vi "Enqueue - ClusterCommand.vi"(5 "Insert? (T)":bool=TRUE, 7 "At Front?":bool, 8 "error in (no error)":errorcluster, 10 "Command":string, 11 "Queue with Cluster Reference":T1) -> (0 "error out":errorcluster, 3 "Queue Out (dup)":T1)   [LabVIEW 2010]
doc: "This VI enqueues only the command portion of the cluster into the referenced queue.\n\nInputs:\nQueue with Cluster Reference - (queue) queue to insert cluster into\nCommand - (string) command part of the cluster to be inserted into the queue (may have arguments)\nAt Front? (F) - (bool) set TRUE to insert cluster at the beginning of the queue; FALSE (default) at the end\nInsert? (T) - (bool) TRUE = insert cluster into queue (default); FALSE = do not insert cluster (controlled via logic)\nerror in - error input cluster\n\nOutputs:\nQueue Out (dup) - (queue) duplicate reference to input queue\nerror out - error output cluster"
uses:
  <userlib>/Common/Queue with Cluster/TYP_Queue with Cluster Reference.ctl
panel:
  # "Inputs"
  # "Outputs"
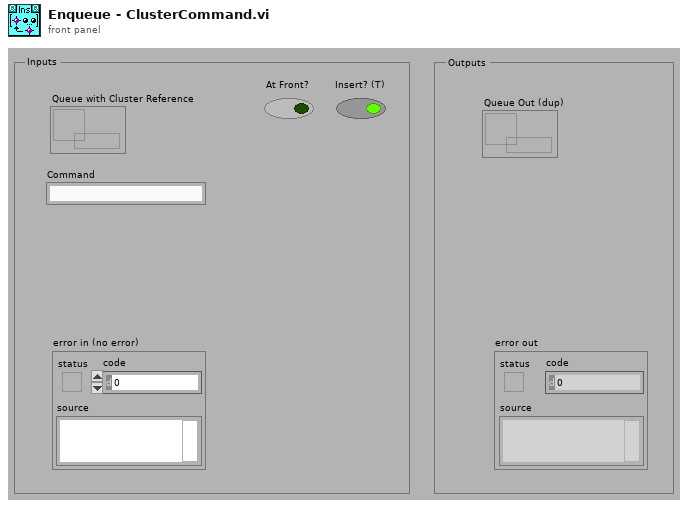
[diagram p1: front panel]
types:
  T1 = typedef "TYP_Queue with Cluster Reference.ctl" = refnum<queue>
  T2 = typedef "TYP_Queue Cluster Element.ctl" = cluster{"Command":string, "Data":variant}
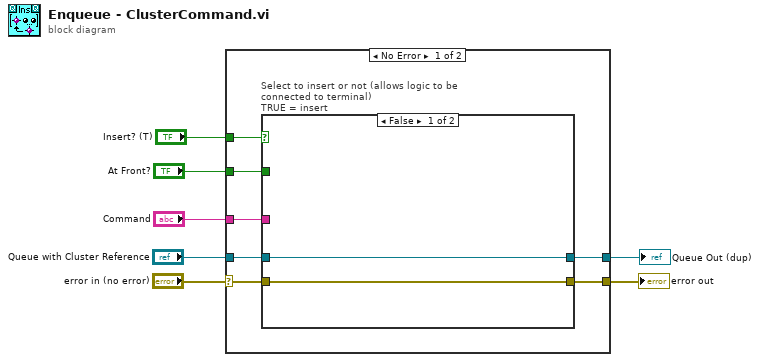
[diagram p0: block diagram]
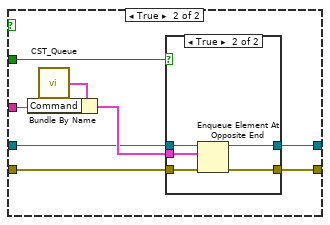
[diagram p2: hidden frame]
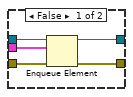
[diagram p3: hidden frame]
diagram:
  n1 = case shown="No Error" "error in (no error)" {
    selector: "error in (no error)" -> [w10 w36]
    tunnel: [w13 w36] -> w6
    tunnel: "Command" -> [w11 _]
    tunnel: "Queue with Cluster Reference" -> [w14 w35]
    tunnel: [w12 w35] -> w3
    tunnel: "At Front?" -> [w9 _]
    tunnel: "Insert? (T)" -> [w8 _]
    frame No Error {
      n2 = case "Select to insert or not (allows logic to be connected to terminal)\nTRUE = insert" shown="False" w8 {
        tunnel: w14 -> [w16 w22]
        tunnel: [w15 w21] -> w13
        tunnel: [w16 w20] -> w12
        tunnel: w11 -> [_ w19]
        tunnel: w10 -> [w15 w18]
        tunnel: w9 -> [_ w17]
        frame False {
        }
        frame True {
          n3 = call <userlib>:"CST_Queue.vi"() -> ("Queue Cluster Element"=w24:T2)  [unwired: 1 in]
          n4 = Bundle By Name(cluster=w24, "Command"=w19) -> (w23:T2)
          n5 = case shown="True" w17 {
            tunnel: w23 -> [w29 w30]
            tunnel: w22 -> [w28 w34]
            tunnel: [w27 w32] -> w21
            tunnel: [w26 w33] -> w20
            tunnel: w18 -> [w25 w31]
            frame False {
              n6 = Enqueue Element(queue=w28, element=w29, error in (no error)=w25) -> (queue out=w26:T1, error out=w27:errorcluster)  [unwired: 1 in, 1 out]
            }
            frame True {
              n7 = Enqueue Element At Opposite End(queue=w34, element=w30, error in (no error)=w31) -> (queue out=w33:T1, error out=w32:errorcluster)  [unwired: 1 in, 1 out]
            }
          }
        }
      }
    }
    frame Error {
    }
  }
  "error out" <- w6
  "Queue Out (dup)" <- w3
